vi "get acceptance level.vi"(0 "IMAQ OCR Session":T1) -> (2 "IMAQ OCR Session (dup)":T1, 4 "error out 3":errorcluster)   [LabVIEW 2011]
uses:
  <vilib>/vision/OCR.llb/IMAQ OCR Property.ctl
  <vilib>/vision/OCR.llb/IMAQ OCR Session.ctl
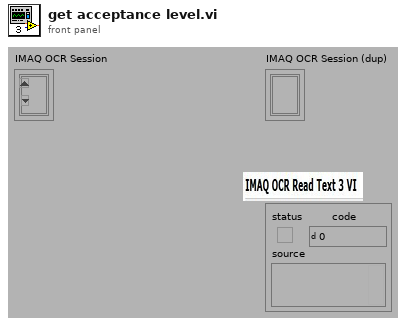
[diagram p1: front panel]
types:
  T1 = typedef "IMAQ OCR Session.ctl" = refnum<k1>
  T2 = typedef "IMAQ OCR Property.ctl" = i32
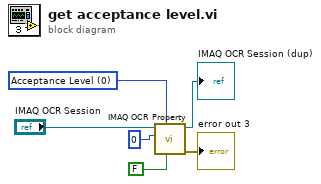
[diagram p0: block diagram]
diagram:
  w5 = T2 0 items=["Acceptance Level", "Min Char Size", "Max Char Size", "Min Char Spacing", "Max Horiz Element Spacing", "Max Vert Element Spacing", "Min Bounding Rect Width", "Max Bounding Rect Width", "Min Bounding Rect Height", "Max Bounding Rect Height", "Read Strategy", "Aspect Ratio", "Number Of Erosions", "Read Resolution", "Size of Char Set", "Substitution Character", "Remove Particles Touching ROI", "Auto Split", "Threshold Type", "Text Detection", "Line Separator", "Shortest Path Segment", "Min Pixels for Space"] ("Property")
  n1 = call-poly "IMAQ OCR Property"("Get/Set (True: Set)"=FALSE, "Property"=w5, "Property Value"=0, "IMAQ OCR Session"="IMAQ OCR Session") -> ("error out"=→"error out 3":errorcluster, "IMAQ OCR Session (dup)"=→"IMAQ OCR Session (dup)":T1)  [unwired: 5 in, 1 out]
